vi "Resolve Template Variable.vi"(8 "error in (no error)":errorcluster, 10 "Variable Name":string, 11 "TemplateVariableResolver in":refnum<class "TemplateVariableResolver.lvclass">) -> (0 "error out":errorcluster, 2 "Value":string)   [LabVIEW 2020, in "HTTP Server.lvlib" / "TemplateVariableResolver.lvclass"]
uses:
  TemplateVariableResolver.lvclass
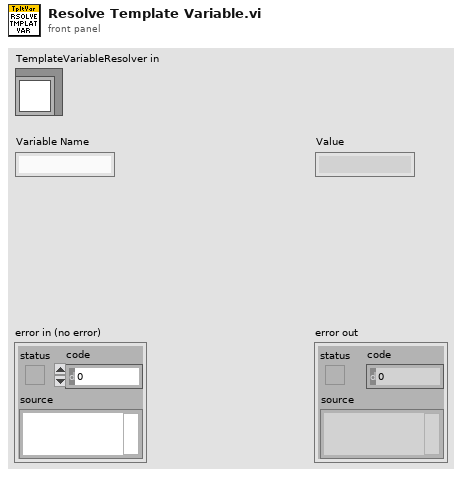
[diagram p1: front panel]
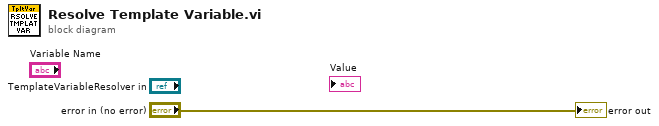
[diagram p0: block diagram]
diagram:
  "error out" <- "error in (no error)"
